vi "Read Paquetes disponibles.vi"(8 "error in (no error)":errorcluster, 11 "Paquetes Disponibles in":refnum<class "Paquetes Disponibles.lvclass">) -> (0 "error out":errorcluster, 2 "Paquetes disponibles":refnum<vi>, 3 "Paquetes Disponibles out":refnum<class "Paquetes Disponibles.lvclass">)   [LabVIEW 2020, in "Paquetes Disponibles.lvlib" / "Paquetes Disponibles.lvclass"]
uses:
  Paquetes Disponibles.lvclass
  Paquetes Disponibles.lvclass/Paquetes Disponibles.ctl
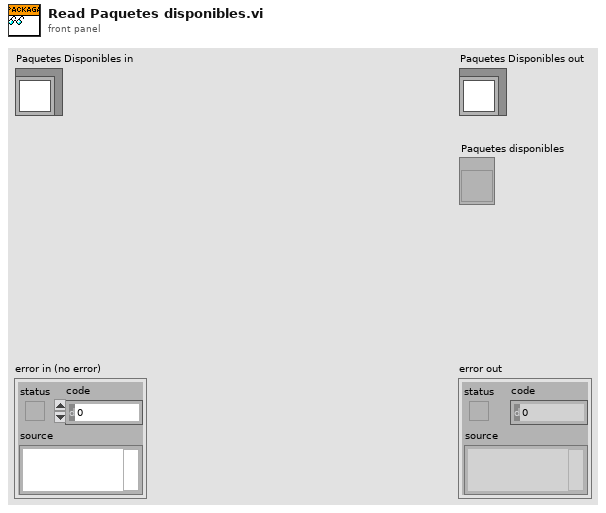
[diagram p1: front panel]
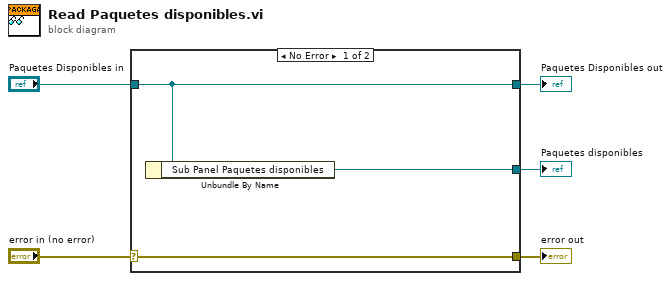
[diagram p0: block diagram]
diagram:
  n1 = case shown="No Error" "error in (no error)" {
    selector: "error in (no error)" -> [w8 w9]
    tunnel: [w8 w9] -> w4
    tunnel: [w7 w10] -> w2
    tunnel: "Paquetes Disponibles in" -> [w7 w10]
    tunnel: [w6 _] -> w1
    frame No Error {
      n2 = Unbundle By Name(w7) -> ("Sub Panel Paquetes disponibles"=w6:refnum<vi>)
    }
    frame Error {
    }
  }
  "error out" <- w4
  "Paquetes Disponibles out" <- w2
  "Paquetes disponibles" <- w1
